vi "tkrsa6100 Initialize.vi"(0 "VISA Resource Name":refnum<visa-resource-name>, 5 "Preset? (Yes)":enum16{"YES", "NO"}(ring), 7 "ID Inst? (Yes)":enum16{"YES", "NO"}(ring), 11 "error in (no error)":errorcluster {"code" format="%#.0f"}) -> (4 "dup VISA Resource Name":refnum<visa-resource-name>, 6 "*IDN? Response":string, 8 "RSA6106A?":bool, 10 "RSA6114A?":bool, 15 "error out":errorcluster {"code" format="%#.0f"})   [LabVIEW 2020, in "Library Instrument & Equipement.lvlib" / "Library Spectrum Analyser.lvlib"]
doc: "This VI opens a VISA Resource Name and if desired, performs a *RST reset and/or an instrument *IDN? query.\n\nThe user inputs a VISA name string in the form <GPIB port #>::<GPIB Address>::INSTR (i.e. GPIB0::1::INSTR). This example corresponds to GPIB Port 0 and instrument GPIB address 1.\n\nThe VISA name string is passed to the VISA Open function along with the error out cluster. The VISA Open function generates VISA Resource Name which is passed to an INSTR Property Node which sets the following:\n\nGPIB Timeout is set to 10S (10000ms)\n\nBased on the setting of the Preset? enumerated control, an *RST command may be sent to the instrument.\n\nBased on the setting of the ID Inst? enumerated control, an IDN? query may be sent to the instrument. The insrument response to the query appears in *IDN? Response string indicator. *IDN? Response String is tested for RSA6106A or RSA6114A and the appropriate boolean indicator is set to TRUE to indicate the instrument type.\n\nThe error out status indicator is then checked for any error condition. If an error has occured, the VISA Resource Name is closed and the error informaton is returned to the calling function in error out. \n\nIf an error has not occured the VI terminates and dup VISA Resource Name, error out (with no error detected), and *IDN? Response are passed back to the calling function."
uses:
  Library Spectrum Analyser.lvlib
panel:
  out "RSA5126?":bool
  out "RSA5115?":bool
  out "RSA6120A?":bool
  out "RSA5103A?":bool
  out "RSA5106A?":bool
  # "RSA6100 Initialize Driver"
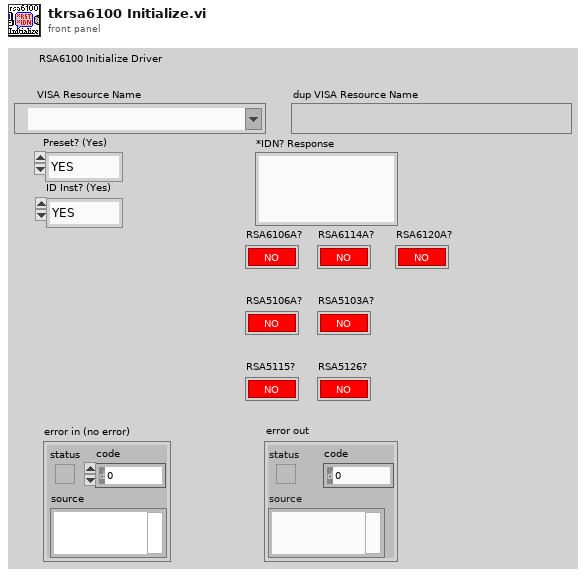
[diagram p1: front panel]
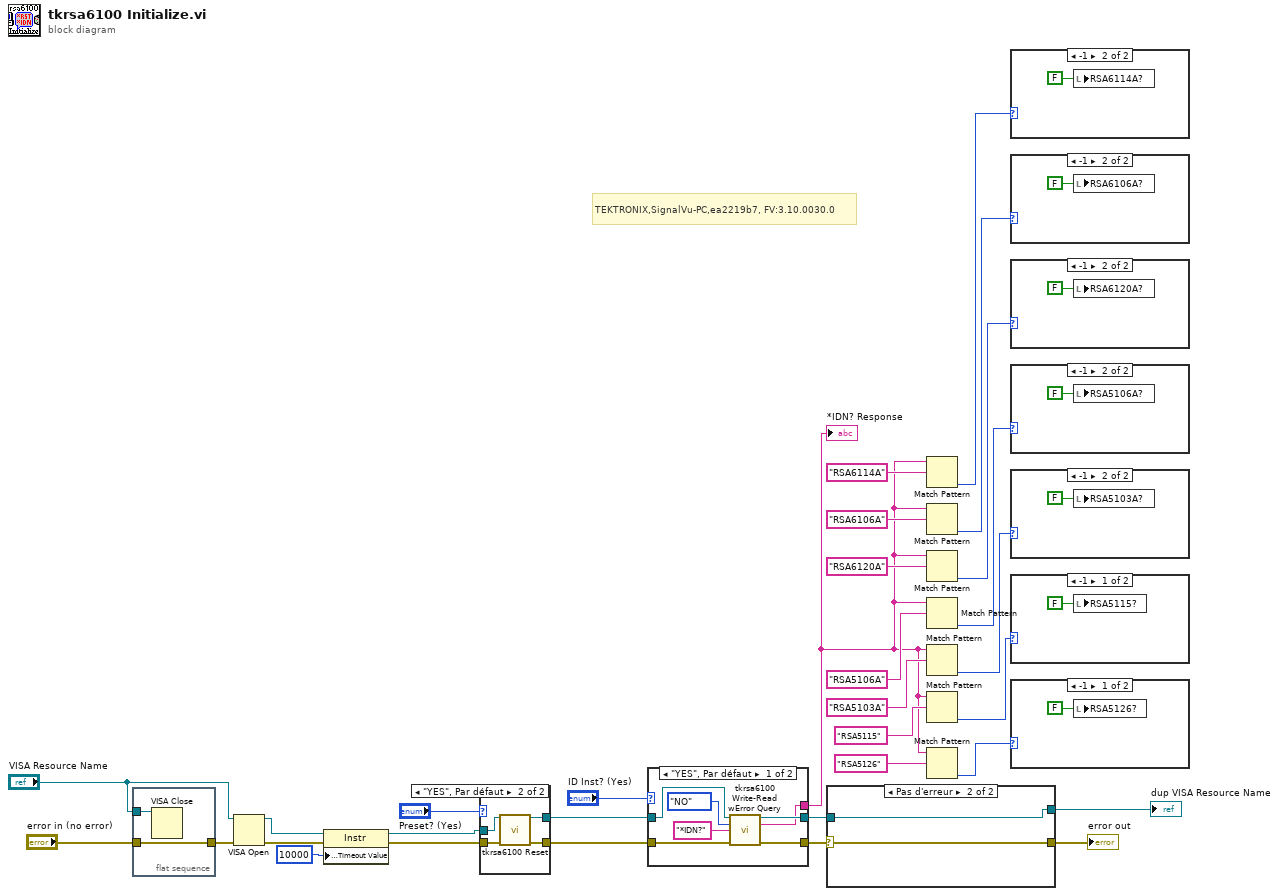
[diagram p0: block diagram]
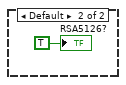
[diagram p2: hidden frame]
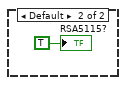
[diagram p3: hidden frame]
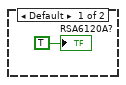
[diagram p4: hidden frame]
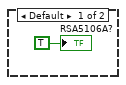
[diagram p5: hidden frame]
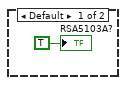
[diagram p6: hidden frame]
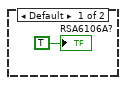
[diagram p7: hidden frame]
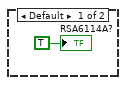
[diagram p8: hidden frame]
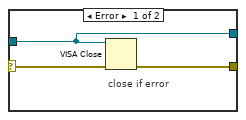
[diagram p9: hidden frame]
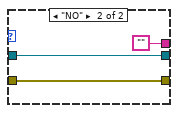
[diagram p11: hidden frame]
diagram:
  # "TEKTRONIX,SignalVu-PC,ea2219b7, FV:3.10.0030.0"
  n1 = flat-sequence {
    tunnel: "VISA Resource Name" -> [w33]
    tunnel: [w32] -> w2
    tunnel: "error in (no error)" -> [w32]
    frame #0 {
      n2 = VISA Close(VISA resource name=w33) -> ()  [unwired: 1 in, 1 out]
    }
  }
  n3 = VISA Open(error in (no error)=w2, VISA resource name="VISA Resource Name") -> (VISA resource name=w27:refnum<visa-resource-name>, error out=w21:errorcluster)  [unwired: 1 in, 2 out]
  n4 = property class="Instr"(reference=w27, error in=w21, "General Settings:Timeout Value"=u32 10000) -> (reference out=w29:refnum<visa-resource-name>, error out=w31:errorcluster)
  n5 = case shown="\"YES\", Par défaut" "Preset? (Yes)" {
    tunnel: w31 -> [w35 w36]
    tunnel: [w35 w39] -> w30
    tunnel: w29 -> [w34 w37]
    tunnel: [w34 w38] -> w28
    frame "NO" {
    }
    frame "YES", Default {
      n6 = call "tkrsa6100 Reset.vi"("VISA Resource Name"=w37, "error in (no error)"=w36) -> ("dup VISA Resource Name"=w38:refnum<visa-resource-name>, "error out"=w39:errorcluster)  [unwired: 12 out]
    }
  }
  n7 = case shown="\"YES\", Par défaut" "ID Inst? (Yes)" {
    tunnel: w28 -> [w46 w49]
    tunnel: w30 -> [w45 w48]
    tunnel: [w42 w48] -> w20
    tunnel: [w43 w49] -> w25
    tunnel: [w41 ""] -> w4
    frame "YES", Default {
      n8 = call "tkrsa6100 Write-Read wError Query.vi"("VISA Resource Name"=w46, "Error Query(YES)"=enum16{"NO", "YES"}."NO", "Command (Empty String)"="*IDN?" ("write buffer (\"\")"), "error in (no error)"=w45) -> ("dup VISA Resource Name"=w43:refnum<visa-resource-name>, "Response"=w41:string, "error out"=w42:errorcluster)  [unwired: 3 in, 6 out]
    }
    frame "NO" {
    }
  }
  "*IDN? Response" <- w4
  n9 = case shown="Pas d'erreur" w20 {
    selector: w20 -> [w50 w53]
    tunnel: w25 -> [w51 w54]
    tunnel: [w52 w53] -> w26
    tunnel: [w51 w54] -> w19
    frame Error {
      # "close if error"
      n10 = VISA Close(VISA resource name=w51, error in (no error)=w50) -> (error out=w52:errorcluster)
    }
    frame No Error {
    }
  }
  "error out" <- w26
  "dup VISA Resource Name" <- w19
  n11 = Match Pattern(string=w4, regular expression="RSA6114A") -> (offset past match=w15:i32)  [unwired: 4 out]
  n12 = Match Pattern(string=w4, regular expression="RSA6106A") -> (offset past match=w16:i32)  [unwired: 4 out]
  n13 = Match Pattern(string=w4, regular expression="RSA6120A") -> (offset past match=w10:i32)  [unwired: 4 out]
  n14 = Match Pattern(string=w4, regular expression="RSA5106A") -> (offset past match=w14:i32)  [unwired: 4 out]
  n15 = Match Pattern(string=w4, regular expression="RSA5103A") -> (offset past match=w12:i32)  [unwired: 4 out]
  n16 = Match Pattern(string=w4, regular expression="RSA5115") -> (offset past match=w8:i32)  [unwired: 4 out]
  n17 = Match Pattern(string=w4, regular expression="RSA5126") -> (offset past match=w5:i32)  [unwired: 4 out]
  n18 = case shown="-1" w15 {
    frame Default {
      "RSA6114A?" <- TRUE ("RSA6114A?")
    }
    frame -1 {
      n19 = local write "RSA6114A?"(FALSE ("RSA6114A?")) -> ()
    }
  }
  n20 = case shown="-1" w16 {
    frame Default {
      "RSA6106A?" <- TRUE ("RSA6114A?")
    }
    frame -1 {
      n21 = local write "RSA6106A?"(FALSE ("RSA6114A?")) -> ()
    }
  }
  n22 = case shown="-1" w10 {
    frame Default {
      "RSA6120A?" <- TRUE ("RSA6114A?")
    }
    frame -1 {
      n23 = local write "RSA6120A?"(FALSE ("RSA6114A?")) -> ()
    }
  }
  n24 = case shown="-1" w14 {
    frame Default {
      "RSA5106A?" <- TRUE ("RSA6114A?")
    }
    frame -1 {
      n25 = local write "RSA5106A?"(FALSE ("RSA6114A?")) -> ()
    }
  }
  n26 = case shown="-1" w12 {
    frame Default {
      "RSA5103A?" <- TRUE ("RSA6114A?")
    }
    frame -1 {
      n27 = local write "RSA5103A?"(FALSE ("RSA6114A?")) -> ()
    }
  }
  n28 = case shown="-1" w8 {
    frame -1 {
      n29 = local write "RSA5115?"(FALSE ("RSA6114A?")) -> ()
    }
    frame Default {
      "RSA5115?" <- TRUE ("RSA6114A?")
    }
  }
  n30 = case shown="-1" w5 {
    frame -1 {
      n31 = local write "RSA5126?"(FALSE ("RSA6114A?")) -> ()
    }
    frame Default {
      "RSA5126?" <- TRUE ("RSA6114A?")
    }
  }
